vi "mapping.vi"(7 "in":dbl, 8 "maxOut":dbl, 9 "minOut":dbl, 10 "maxIn":dbl, 11 "minIn":dbl) -> (3 "out":dbl)   [LabVIEW 2017]
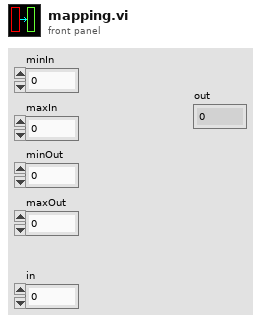
[diagram p1: front panel]
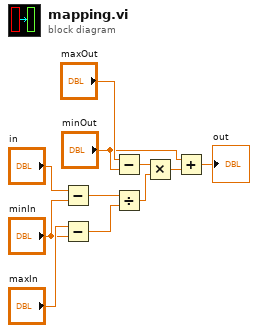
[diagram p0: block diagram]
diagram:
  n1 = Subtract(x="in", y="minIn") -> (x-y=w8:dbl)
  n2 = Subtract(x="maxIn", y="minIn") -> (x-y=w7:dbl)
  n3 = Subtract(x="maxOut", y="minOut") -> (x-y=w5:dbl)
  n4 = Divide(x=w8, y=w7) -> (x/y=w4:dbl)
  n5 = Multiply(x=w5, y=w4) -> (x*y=w2:dbl)
  n6 = Add(x="minOut", y=w2) -> (x+y=→"out":dbl)
